vi "BRig_RT__Case_Idle__State_RewardCalibration.vi"(7 "input_state":T1, 11 "input_dataMTrig":u16[](array[numeric])) -> (3 "output_dataMtrig":u16[](array[numeric]), 5 "output_state":T1)   [LabVIEW 2014]
uses:
  myRIO_BRig_RT__Case_NonExp_stateList.ctl
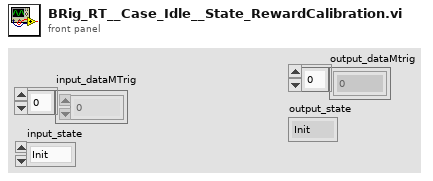
[diagram p1: front panel]
types:
  T1 = typedef "myRIO_BRig_RT__Case_NonExp_stateList.ctl" = enum16{"Init", "UploadSettings_pre", "UploadSettings_Read_dataExp", "UploadSettings_dataExp_1", "UploadSettings_dataExp_2", "UploadSettings_Read_dataLC", "UploadSettings_dataLC_1", "UploadSettings_dataLC_2", "UploadSettings_dataLC_3", "UploadSettings_dataLC_4", "UploadSettings_Read_dataMTrig", "UploadSettings_dataMTrig_1", "UploadSettings_post", "Idle_pre", "IdleEmpty", "IdleEmpty2", "IdleEmpty3", "IdleEmpty4", "Idle", "Idle_2", "Idle_3", "Idle_4", "Idle_5", "Idle_6", "Idle_post", "Cue_pre__pre", "Cue_pre", "Cue", "Cue_LED", "Cue_post", "RewardCalibration_pre", "RewardCalibration", "DispenseWater_pre__pre", "DispenseWater_pre", "DispenseWater", "DispenseWater_post", "TestConnection", "SendData", "Get_FPGA_count_per_ms", "End", "commTCP_connect"}
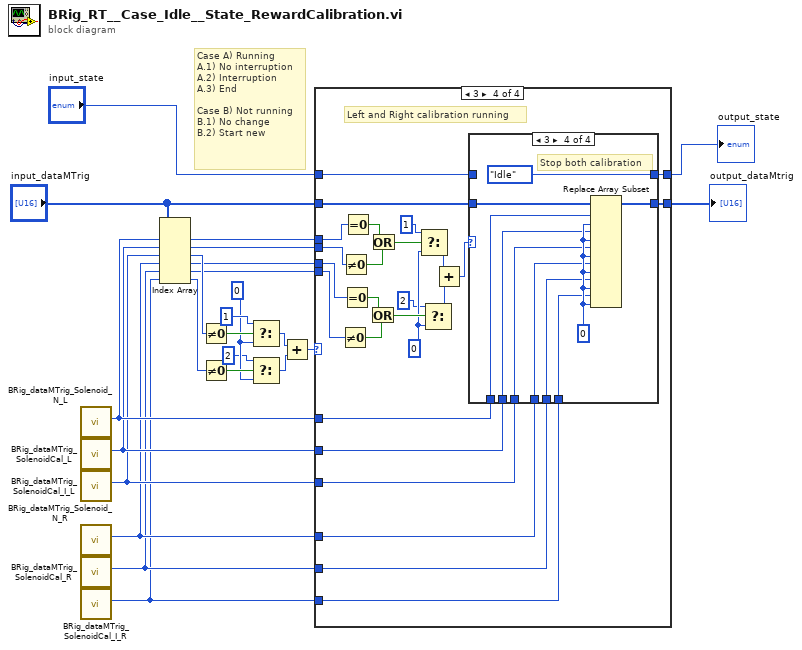
[diagram p0: block diagram]
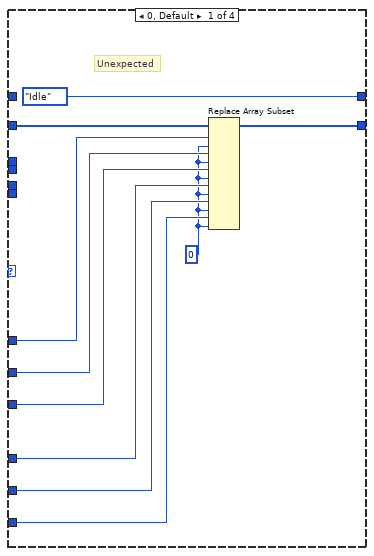
[diagram p2: hidden frame]
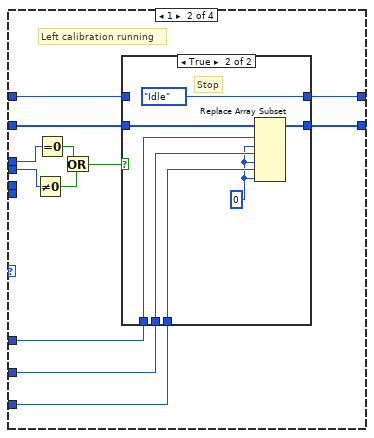
[diagram p3: hidden frame]
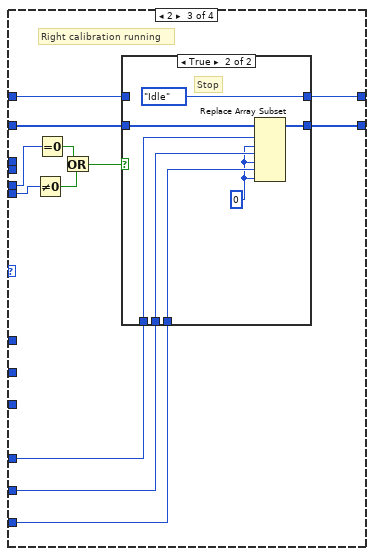
[diagram p5: hidden frame]
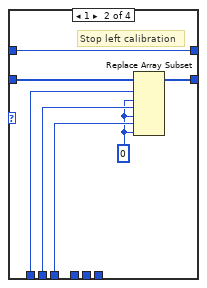
[diagram p8: hidden frame]
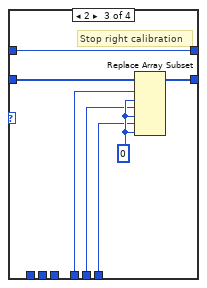
[diagram p9: hidden frame]
diagram:
  w19 = 0 ("f")
  # "Case A) Running\nA.1) No interruption\nA.2) Interruption\nA.3) End\n\nCase B) Not running\nB.1) No change\nB.2) Start new"
  n1 = call "BRig_dataMTrig_Solenoid_N_L.vi"() -> ("output_Solenoid_N_L"=w9:i32)  [unwired: 11 in]
  n2 = call "BRig_dataMTrig_SolenoidCal_L.vi"() -> ("output_SolenoidCal_L"=w8:i32)  [unwired: 11 in]
  n3 = call "BRig_dataMTrig_SolenoidCal_I_L.vi"() -> ("output_SolenoidCal_I_L"=w7:i32)  [unwired: 11 in]
  n4 = call "BRig_dataMTrig_Solenoid_N_R.vi"() -> ("output_Solenoid_N_R"=w6:i32)  [unwired: 11 in]
  n5 = call "BRig_dataMTrig_SolenoidCal_R.vi"() -> ("output_SolenoidCal_R"=w5:i32)  [unwired: 11 in]
  n6 = call "BRig_dataMTrig_SolenoidCal_I_R.vi"() -> ("output_SolenoidCal_I_R"=w4:i32)  [unwired: 11 in]
  n7 = Index Array(array="input_dataMTrig", index #1=w9, index #2=w8, index #3=w7, index #4=w6, index #5=w5, index #6=w4) -> (element #1=w14:u16, element #2=w13:u16, element #3=w24:u16, element #4=w12:u16, element #5=w11:u16, element #6=w20:u16)
  n8 = Not Equal To 0?(x=w24) -> (x != 0?=w23:bool)
  n9 = Not Equal To 0?(x=w20) -> (x != 0?=w21:bool)
  n10 = Select(t=1, s=w23, f=w19) -> (s? t:f=w17:i32)
  n11 = Select(t=2, s=w21, f=w19) -> (s? t:f=w16:i32)
  n12 = Add(x=w17, y=w16) -> (x+y=w15:i32)
  n13 = case shown="3" w15 {
    tunnel: w14 -> [_ w45 _ w101]
    tunnel: w13 -> [_ w46 _ w102]
    tunnel: w12 -> [_ _ w57 w92]
    tunnel: w11 -> [_ _ w56 w91]
    tunnel: "input_dataMTrig" -> [w33 w41 w64 w98]
    tunnel: [myRIO_BRig_RT__Case_NonExp_stateList."Idle" ("Enum") w39 w62 w96] -> w1
    tunnel: [w32 w38 w61 w95] -> w10
    tunnel: "input_state" -> [_ w40 w63 w97]
    tunnel: w9 -> [w31 w37 _ w82]
    tunnel: w8 -> [w30 w36 _ w81]
    tunnel: w7 -> [w29 w35 _ w80]
    tunnel: w6 -> [w28 _ w60 w79]
    tunnel: w5 -> [w27 _ w59 w78]
    tunnel: w4 -> [w26 _ w58 w77]
    frame 0, Default {
      w25 = u16 0 ("new element/subarray")
      # "Unexpected"
      n14 = Replace Array Subset(array=w33, new element #1=w25, index #1=w31, new element #2=w25, index #2=w30, new element #3=w25, index #3=w29, new element #4=w25, index #4=w28, new element #5=w25, index #5=w27, new element #6=w25, index #6=w26) -> (w32:u16[])
    }
    frame 1 {
      # "Left calibration running"
      n15 = Not Equal To 0?(x=w46) -> (x != 0?=w43:bool)
      n16 = Equal To 0?(x=w45) -> (x = 0?=w44:bool)
      n17 = Or(x=w44, y=w43) -> (x .or. y?=w42:bool)
      n18 = case shown="True" w42 {
        tunnel: w41 -> [w47 w53]
        tunnel: w40 -> [w48 _]
        tunnel: [w48 myRIO_BRig_RT__Case_NonExp_stateList."Idle" ("Enum")] -> w39
        tunnel: [w47 w54] -> w38
        tunnel: w37 -> [_ w52]
        tunnel: w36 -> [_ w51]
        tunnel: w35 -> [_ w50]
        frame False {
        }
        frame True {
          w49 = u16 0 ("new element/subarray")
          # "Stop"
          n19 = Replace Array Subset(array=w53, new element #1=w49, index #1=w52, new element #2=w49, index #2=w51, new element #3=w49, index #3=w50) -> (w54:u16[])
        }
      }
    }
    frame 2 {
      # "Right calibration running"
      n20 = Not Equal To 0?(x=w56) -> (x != 0?=w66:bool)
      n21 = Equal To 0?(x=w57) -> (x = 0?=w67:bool)
      n22 = Or(x=w67, y=w66) -> (x .or. y?=w65:bool)
      n23 = case shown="True" w65 {
        tunnel: w64 -> [w68 w74]
        tunnel: w63 -> [w69 _]
        tunnel: [w69 myRIO_BRig_RT__Case_NonExp_stateList."Idle" ("Enum")] -> w62
        tunnel: [w68 w75] -> w61
        tunnel: w60 -> [_ w73]
        tunnel: w59 -> [_ w72]
        tunnel: w58 -> [_ w71]
        frame False {
        }
        frame True {
          w70 = u16 0 ("new element/subarray")
          # "Stop"
          n24 = Replace Array Subset(array=w74, new element #1=w70, index #1=w73, new element #2=w70, index #2=w72, new element #3=w70, index #3=w71) -> (w75:u16[])
        }
      }
    }
    frame 3 {
      w85 = u8 0
      # "Left and Right calibration running"
      n25 = Not Equal To 0?(x=w91) -> (x != 0?=w94:bool)
      n26 = Not Equal To 0?(x=w102) -> (x != 0?=w99:bool)
      n27 = Equal To 0?(x=w92) -> (x = 0?=w93:bool)
      n28 = Equal To 0?(x=w101) -> (x = 0?=w100:bool)
      n29 = Or(x=w93, y=w94) -> (x .or. y?=w87:bool)
      n30 = Or(x=w100, y=w99) -> (x .or. y?=w90:bool)
      n31 = Select(t=u8 1, s=w90, f=w85) -> (s? t:f=w89:u8)
      n32 = Select(t=u8 2, s=w87, f=w85) -> (s? t:f=w86:u8)
      n33 = Add(x=w89, y=w86) -> (x+y=w88:u8)
      n34 = case shown="3" w88 {
        tunnel: w98 -> [w104 w110 w117 w127]
        tunnel: w97 -> [w103 w105 w115 _]
        tunnel: [w103 w105 w115 myRIO_BRig_RT__Case_NonExp_stateList."Idle" ("Enum")] -> w96
        tunnel: [w104 w111 w118 w128] -> w95
        tunnel: w82 -> [_ w109 _ w119]
        tunnel: w81 -> [_ w108 _ w120]
        tunnel: w80 -> [_ w107 _ w121]
        tunnel: w79 -> [_ _ w114 w122]
        tunnel: w78 -> [_ _ w113 w123]
        tunnel: w77 -> [_ _ w112 w124]
        frame 0, Default {
        }
        frame 1 {
          w106 = u16 0 ("new element/subarray")
          # "Stop left calibration"
          n35 = Replace Array Subset(array=w110, new element #1=w106, index #1=w109, new element #2=w106, index #2=w108, new element #3=w106, index #3=w107) -> (w111:u16[])
        }
        frame 2 {
          w116 = u16 0 ("new element/subarray")
          # "Stop right calibration"
          n36 = Replace Array Subset(array=w117, new element #1=w116, index #1=w114, new element #2=w116, index #2=w113, new element #3=w116, index #3=w112) -> (w118:u16[])
        }
        frame 3 {
          w125 = u16 0 ("new element/subarray")
          # "Stop both calibration"
          n37 = Replace Array Subset(array=w127, new element #1=w125, index #1=w119, new element #2=w125, index #2=w120, new element #3=w125, index #3=w121, new element #4=w125, index #4=w122, new element #5=w125, index #5=w123, new element #6=w125, index #6=w124) -> (w128:u16[])
        }
      }
    }
  }
  "output_dataMtrig" <- w10
  "output_state" <- w1
